vi "Template.vi"() -> ()   [LabVIEW 2009]
panel:
  in  "OK Button 4":bool
  in  "OK Button 3":bool
  in  "OK Button 2":bool
  in  "OK Button":bool
  in  "OK Button":bool
  in  "Tab Control":T1(tab)
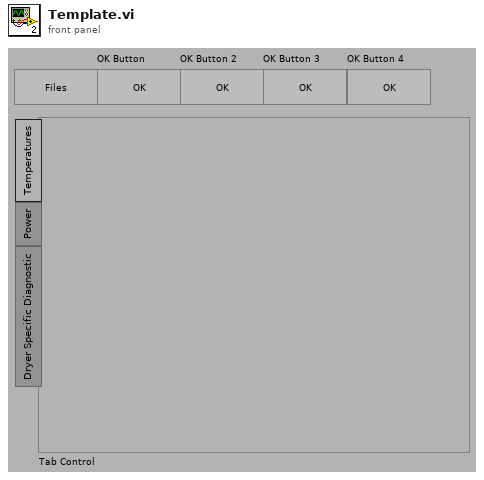
[diagram p1: front panel]
types:
  T1 = enum32{"Temperatures", "Power", "Dryer Specific Diagnostic"}
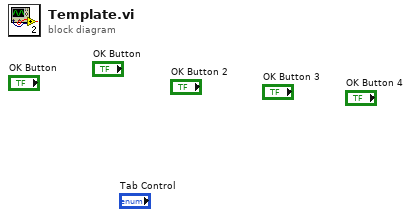
[diagram p0: block diagram]
diagram:
